vi "ex7-3.vi"   [LabVIEW 2013]
uses:
  <vilib>/NXT/Dual Mode Library/Display/drawNumber.vi
  <vilib>/NXT/Dual Mode Library/Waits/Wait_Num.vi
types:
  T1 = typedef "LVHSConnector.ctl" = refnum<class "BrickReference.lvclass">
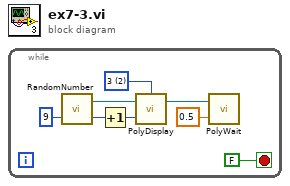
[diagram p0: block diagram]
diagram:
  n1 = while {
    stop <- FALSE stop-if-true
    w4 = i16 2 items=["1", "2", "3", "4", "5", "6", "7", "8", "9", "10", "11", "12"] ("Line")
    n2 = call <vilib>:"RandomNumber.vi"("Max Value"=u16 9) -> ("Random Number"=w3:u16, "NXT"=w6:T1)  [unwired: 2 in]
    n3 = Increment(x=w3) -> (x+1=w2:u16)
    n4 = call-poly <vilib>:"PolyDisplay.vi"("number"=w2, "NXT/EV3"=w6, "Line"=w4) -> ("NXT/EV3"=w5:T1)  [unwired: 1 in]
    n5 = call-poly <vilib>:"PolyWait.vi"("Time (1 sec)"=sgl 0.5, "NXT/EV3"=w5) -> ()  [unwired: 2 in, 1 out]
  }
